vi "Query_MP.vi"(5 "buffered":bool=TRUE, 6 "commandTimeout":i32=-1, 7 "CommandType":i32(ring)=-1 items=["Text"=1, "StoredProcedure"=4, "TableDirect"=512], 8 "error in (no error)":errorcluster, 9 "DynamicParameters":refnum<class "DynamicParameters.lvclass">[](array[class]), 10 "sql":string, 11 "ADOMapper in":refnum<class "ADOMapper.lvclass">) -> (0 "error out":errorcluster, 2 "Query Result out":refnum<class "Query Result.lvclass">, 3 "ADOMapper out":refnum<class "ADOMapper.lvclass">)   [LabVIEW 2020, in "ORM_ADONet.lvlib" / "ADOMapper.lvclass"]
uses:
  ADOMapper.lvclass
  C:/Program Files/National Instruments/LabVIEW 2020/vi.lib/Viviota/shared/ORM.lvlibp/ORM/SqlMapper/SqlMapper.lvclass
  <vilib>/Viviota/shared/ORM.lvlibp/ORM/Query Result/Query Result.lvclass
  <vilib>/Viviota/shared/ORM.lvlibp/ORM/DynamicParameters/DynamicParameters.lvclass
  System.Data
  ADOResult/ADOResult.lvclass
  C:/Program Files/National Instruments/LabVIEW 2020/vi.lib/Viviota/shared/ORM.lvlibp/ORM/Query Result/Query Result.lvclass
  <vilib>/Viviota/shared/ORM.lvlibp/ORM/SqlMapper/Read DbConnection.vi
  <vilib>/Viviota/shared/ORM.lvlibp/ORM/DbConnection/Read transaction.vi
  <vilib>/Viviota/shared/ORM.lvlibp/ORM/DbConnection/DbConnection.lvclass
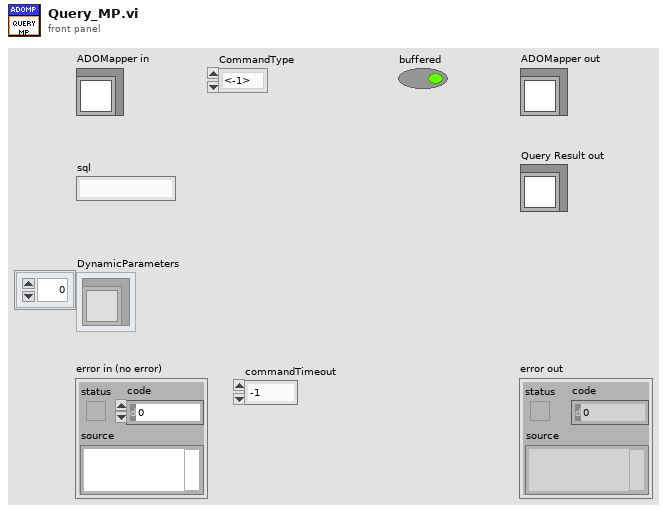
[diagram p1: front panel]
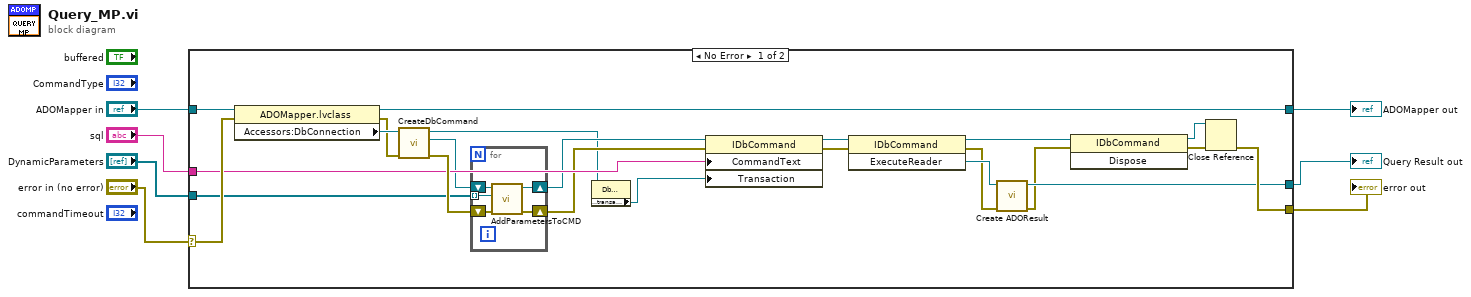
[diagram p0: block diagram]
diagram:
  n1 = case shown="No Error" "error in (no error)" {
    selector: "error in (no error)" -> [w27 w37]
    tunnel: "ADOMapper in" -> [w30 w36]
    tunnel: [w29 w36] -> w6
    tunnel: "sql" -> [w24 _]
    tunnel: [w18 w37] -> w1
    tunnel: "DynamicParameters" -> [w15 _]
    tunnel: [w13 _] -> w5
    frame No Error {
      n2 = property class="ADOMapper.lvclass"(reference=w30, error in=w27) -> (reference out=w29:refnum<class "ADOMapper.lvclass">, error out=w26:errorcluster, "Accessors:DbConnection"=w28:refnum<class "DbConnection.lvclass">)
      n3 = call <vilib>:"CreateDbCommand.vi"("error in (no error)"=w26, "DbConnection in"=w28) -> ("error out"=w25:errorcluster, "CreateCommand"=w16:refnum<k24>, "DbConnection out"=w9:refnum<class "DbConnection.lvclass">)  [unwired: 7 in]
      n4 = for {
        tunnel: w15 -> [w32] mode=indexing
        shift-right: [w34] -> w22
        shift-left: w25 -> [w35]
        shift-right: [w31] -> w14
        shift-left: w16 -> [w33]
        n5 = call "AddParametersToCMD.vi"("error in (no error)"=w35, "DynamicParameters in"=w32, "CreateCommand"=w33) -> ("error out"=w34:errorcluster, "CreateCommand Out"=w31:refnum<k24>)  [unwired: 7 in]
      }
      n6 = property class="DbConnection.lvclass"(reference=w9) -> ("Accessors:transaction"=w8:refnum<k24>)  [unwired: 1 in, 2 out]
      n7 = property class="IDbCommand"(reference=w14, error in=w22, "CommandText"=w24, "Transaction"=w8) -> (reference out=w23:refnum<k24>, error out=w21:errorcluster)
      n8 = invoke class="IDbCommand" method="ExecuteReader"(reference=w23, error in=w21) -> (reference out=w20:refnum<k24>, error out=w11:errorcluster, "ExecuteReader"=w12:refnum<k24>)  [unwired: 1 in]
      n9 = call "Create ADOResult.vi"("error in (no error)"=w11, "Reader"=w12) -> ("error out"=w10:errorcluster, "ADOResult out"=w13:refnum<class "ADOResult.lvclass">)  [unwired: 8 in]
      n10 = invoke class="IDbCommand" method="Dispose"(reference=w20, error in=w10) -> (reference out=w17:refnum<k24>, error out=w19:errorcluster)  [unwired: 1 in, 1 out]
      n11 = Close Reference(reference=w17, error in (no error)=w19) -> (error out=w18:errorcluster)
    }
    frame Error {
    }
  }
  "error out" <- w1
  "ADOMapper out" <- w6
  "Query Result out" <- w5
